vi "nii_write.vi"(7 "datatype":string, 8 "error in (no error)":errorcluster, 9 "data in":cdb[](array[numeric]), 10 "nii_write":path, 11 "nii_source":path) -> (0 "error out":errorcluster)   [LabVIEW 2014]
panel:
  in  "datatype 2":T1(ring)
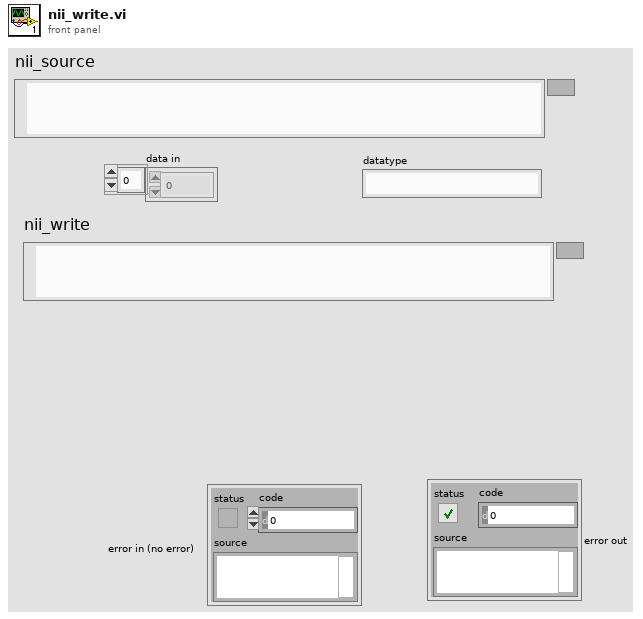
[diagram p1: front panel]
types:
  T1 = enum16{"NONE", "BINARY", "UNSIGNED_CHAR", "SIGNED_SHORT", "SIGNED_INT", "FLOAT", "COMPLEX", "DOUBLE", "RGB", "ALL"}
  T2 = typedef "head_data.ctl" = cluster{"hdr size":i32, "dim":i32[], "data bit size":i32, "datatype":string, "pixel size ":sgl[], "voxel offset":sgl, "range of calibration values-max,min":sgl[], " pixel values- max, min":sgl[], "slice orientation":u16}
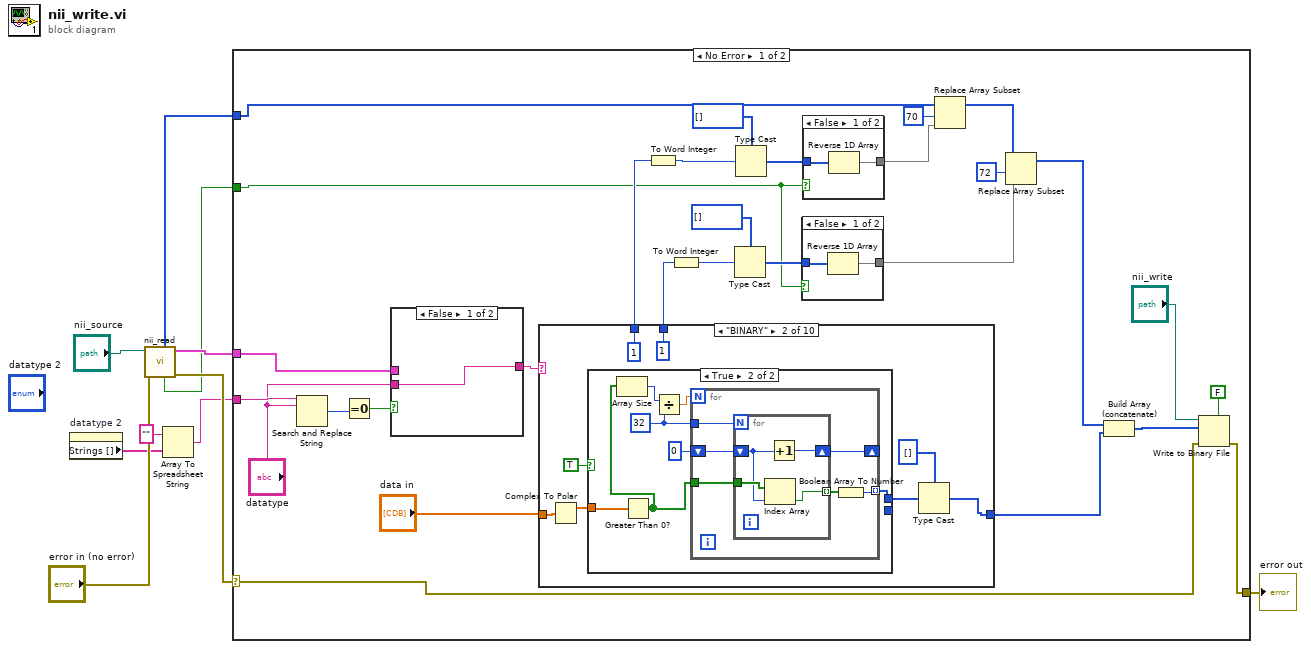
[diagram p0: block diagram]
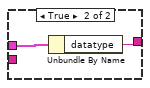
[diagram p4: hidden frame]
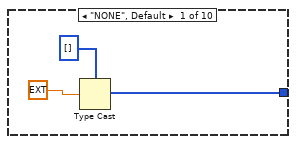
[diagram p5: hidden frame]
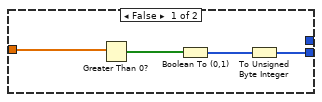
[diagram p6: hidden frame]
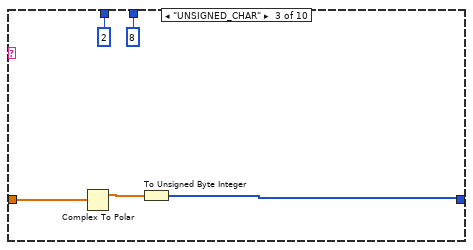
[diagram p7: hidden frame]
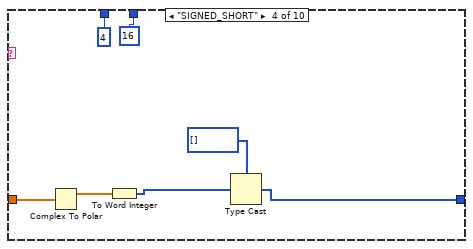
[diagram p8: hidden frame]
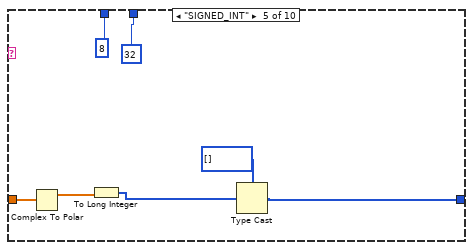
[diagram p9: hidden frame]
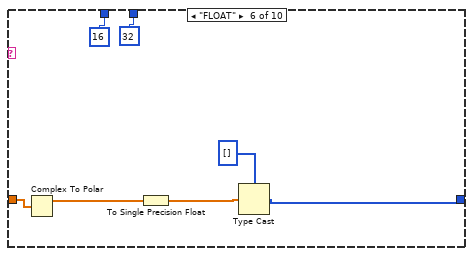
[diagram p10: hidden frame]
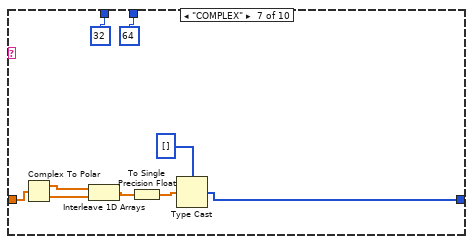
[diagram p11: hidden frame]
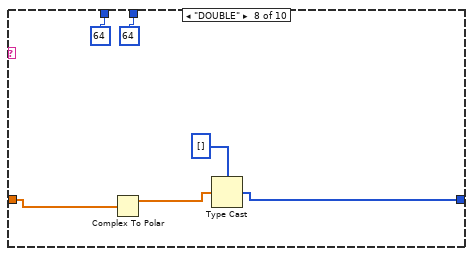
[diagram p12: hidden frame]
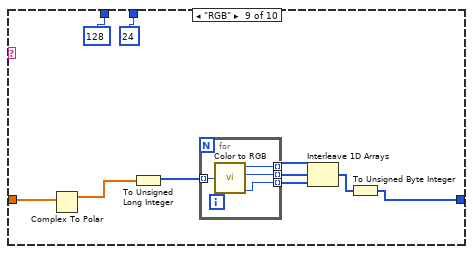
[diagram p13: hidden frame]
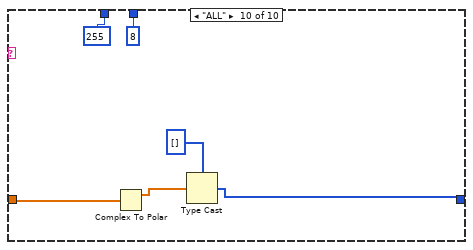
[diagram p14: hidden frame]
diagram:
  n1 = property on="datatype 2" class="Enum (strict)"() -> ("Strings []"=w3:string[])  [unwired: 2 in, 2 out]
  n2 = call "nii_read.vi"("error in (no error)"="error in (no error)", "file (use dialog)"="nii_source") -> ("error out"=w7:errorcluster, "Data"=w9:T2, "non-flip"=w4:bool, "head"=w8:u8[])  [unwired: 5 in, 1 out]
  n3 = Array To Spreadsheet String(array=w3, 3:"" ("format string")) -> (spreadsheet string=w2:string)  [unwired: 1 in]
  n4 = case shown="No Error" w7 {
    selector: w7 -> [w35 w142]
    tunnel: w9 -> [w39 _]
    tunnel: w8 -> [w24 _]
    tunnel: [w34 w142] -> w6
    tunnel: w4 -> [w12 _]
    tunnel: w2 -> [w23 _]
    frame No Error {
      n5 = Search and Replace String(input string=w23, search string="datatype") -> (number of replacements=w20:i32)  [unwired: 6 in, 3 out]
      n6 = Equal To 0?(x=w20) -> (x = 0?=w22:bool)
      n7 = case shown="False" w22 {
        tunnel: w39 -> [_ w48]
        tunnel: [w46 w47] -> w38
        tunnel: "datatype" -> [w46 _]
        frame False {
        }
        frame True {
          n8 = Unbundle By Name(w48) -> ("datatype"=w47:string)
        }
      }
      n9 = case shown="\"BINARY\"" w38 {
        tunnel: [w50 w54 w83 w87 w94 w102 w109 w118 w124 w138] -> w33
        tunnel: "data in" -> [_ w58 w85 w92 w99 w106 w113 w121 w128 w141]
        tunnel: [_ u8 1 u8 2 u8 4 u8 8 u8 16 u8 32 u8 64 u8 128 u8 255] -> w29
        tunnel: [_ u8 1 u8 8 u8 16 u8 32 u8 32 u8 64 u8 64 u8 24 u8 8] -> w11
        frame "NONE", Default {
          n10 = Type Cast(type=u8[] [], x=ext 0.0) -> (*(type *) &x=w50:u8[])
        }
        frame "BINARY" {
          n11 = Complex To Polar(r * e^(i*theta)=w58) -> (r=w57:dbl[])  [unwired: 1 out]
          n12 = case shown="True" TRUE {
            tunnel: w57 -> [w63 w70]
            tunnel: [_ w64] -> w52
            tunnel: [w60 _] -> _
            frame False {
              n13 = Greater Than 0?(x=w63) -> (x > 0?=w62:bool[])
              n14 = Boolean To (0,1)(Boolean=w62) -> (0, 1=w61:i16[])
              n15 = To Unsigned Byte Integer(number=w61) -> (unsigned 8bit integer=w60:u8[])
            }
            frame True {
              w67 = 32
              n16 = Greater Than 0?(x=w70) -> (x > 0?=w65:bool[])
              n17 = Array Size(array=w65) -> (size(s)=w66:i32)
              n18 = Divide(x=w66, y=w67) -> (x/y=w68:dbl)
              n19 = for {
                N: w68 -> [_]
                shift-right: [w76] -> _
                shift-left: 0 -> [w75]
                tunnel: w65 -> [w74]
                tunnel: [w72] -> w64 mode=indexing
                tunnel: w67 -> [w71]
                n20 = for {
                  N: w71 -> [_]
                  shift-right: [w80] -> w76
                  shift-left: w75 -> [w77]
                  tunnel: w74 -> [w79]
                  tunnel: [w78] -> w73 mode=indexing
                  n21 = Index Array(array=w79, index=w77) -> (element=w78:bool)
                  n22 = Increment(x=w77) -> (x+1=w80:i32)
                }
                n23 = Boolean Array To Number(Boolean array=w73) -> (number=w72:u32)
              }
            }
          }
          n24 = Type Cast(type=u8[] [], x=w52) -> (*(type *) &x=w54:u8[])
        }
        frame "UNSIGNED_CHAR" {
          n25 = Complex To Polar(r * e^(i*theta)=w85) -> (r=w84:dbl[])  [unwired: 1 out]
          n26 = To Unsigned Byte Integer(number=w84) -> (unsigned 8bit integer=w83:u8[])
        }
        frame "SIGNED_SHORT" {
          n27 = Complex To Polar(r * e^(i*theta)=w92) -> (r=w91:dbl[])  [unwired: 1 out]
          n28 = To Word Integer(number=w91) -> (16bit integer=w88:i16[])
          n29 = Type Cast(type=u8[] [], x=w88) -> (*(type *) &x=w87:u8[])
        }
        frame "SIGNED_INT" {
          n30 = Complex To Polar(r * e^(i*theta)=w99) -> (r=w98:dbl[])  [unwired: 1 out]
          n31 = To Long Integer(number=w98) -> (32bit integer=w95:i32[])
          n32 = Type Cast(type=u8[] [], x=w95) -> (*(type *) &x=w94:u8[])
        }
        frame "FLOAT" {
          n33 = Complex To Polar(r * e^(i*theta)=w106) -> (r=w105:dbl[])  [unwired: 1 out]
          n34 = To Single Precision Float(number=w105) -> (single precision float=w101:sgl[])
          n35 = Type Cast(type=u8[] [], x=w101) -> (*(type *) &x=w102:u8[])
        }
        frame "COMPLEX" {
          n36 = Complex To Polar(r * e^(i*theta)=w113) -> (r=w115:dbl[], theta=w114:dbl[])
          n37 = Interleave 1D Arrays(w115, w114) -> (w111:dbl[])
          n38 = To Single Precision Float(number=w111) -> (single precision float=w110:sgl[])
          n39 = Type Cast(type=u8[] [], x=w110) -> (*(type *) &x=w109:u8[])
        }
        frame "DOUBLE" {
          n40 = Complex To Polar(r * e^(i*theta)=w121) -> (r=w119:dbl[])  [unwired: 1 out]
          n41 = Type Cast(type=u8[] [], x=w119) -> (*(type *) &x=w118:u8[])
        }
        frame "RGB" {
          n42 = Complex To Polar(r * e^(i*theta)=w128) -> (r=w127:dbl[])  [unwired: 1 out]
          n43 = To Unsigned Long Integer(number=w127) -> (unsigned 32bit integer=w126:u32[])
          n44 = for {
            tunnel: [w135] -> w131 mode=indexing
            tunnel: [w134] -> w130 mode=indexing
            tunnel: [w133] -> w129 mode=indexing
            tunnel: w126 -> [w132] mode=indexing
            n45 = call <vilib>:"Color to RGB.vi"("Color"=w132) -> ("Resolved Color"=w135:u32, "R"=w134:u8, "B"=w133:u8)  [unwired: 1 out]
          }
          n46 = Interleave 1D Arrays(w131, w130, w129) -> (w125:u32[])
          n47 = To Unsigned Byte Integer(number=w125) -> (unsigned 8bit integer=w124:u8[])
        }
        frame "ALL" {
          n48 = Complex To Polar(r * e^(i*theta)=w141) -> (r=w139:dbl[])  [unwired: 1 out]
          n49 = Type Cast(type=u8[] [], x=w139) -> (*(type *) &x=w138:u8[])
        }
      }
      n50 = To Word Integer(number=w29) -> (16bit integer=w27:i16)
      n51 = To Word Integer(number=w11) -> (16bit integer=w15:i16)
      n52 = Type Cast(type=u8[] [], x=w15) -> (*(type *) &x=w16:u8[])
      n53 = Type Cast(type=u8[] [], x=w27) -> (*(type *) &x=w26:u8[])
      n54 = case shown="False" w12 {
        tunnel: [w41 w42] -> w13
        tunnel: w16 -> [w40 w42]
        frame False {
          n55 = Reverse 1D Array(array=w40) -> (reversed array=w41:u8[])
        }
        frame True {
        }
      }
      n56 = case shown="False" w12 {
        tunnel: [w44 w45] -> w25
        tunnel: w26 -> [w43 w45]
        frame False {
          n57 = Reverse 1D Array(array=w43) -> (reversed array=w44:u8[])
        }
        frame True {
        }
      }
      n58 = Replace Array Subset(array=w24, new element=w25, index=70) -> (w19:u8[])
      n59 = Replace Array Subset(array=w19, new element=w13, index=72) -> (w17:u8[])
      n60 = Build Array (concatenate)(w17, w33) -> (w32:u8[])
      n61 = Write to Binary File(file (use dialog)="nii_write", data=w32, error in=w35, 5:FALSE ("prepend array or string size? (T)")) -> (error out=w34:errorcluster)  [unwired: 2 in, 2 out]
    }
    frame Error {
    }
  }
  "error out" <- w6
